vi "receive incidents.vi"(7 "queues":T1, 11 "comms in":T2) -> ()   [LabVIEW 2018]
uses:
  type defs/comms loop data.ctl
  ICL-LabVIEW_General/Incident logger/Incident logger.lvclass
  <vilib>/Modbus/master/Modbus Master.lvclass
  type defs/Queues.ctl
  RT/Type Defs/generic incident.ctl
  RT/Type Defs/warning incident cluster.ctl
  RT/Type Defs/error incident cluster.ctl
  ICL-LabVIEW_General/Incident logger/Incidents/Warning/Warning.lvclass
  C:/Users/cnoon/OneDrive - Imperial College London/LabVIEW/Chris VIs/Incident logger/Incidents/Incident.lvclass
  ICL-LabVIEW_General/Incident logger/Incidents/Message/Message.lvclass
  ICL-LabVIEW_General/Incident logger/Incidents/Error/Error.lvclass
  supporting VIs/polymorphic VIs/enqueue for message handler.vi
  <resource>/objmgr/ni.dex.rc
types:
  T1 = typedef "Queues.ctl" = cluster{"messageHandler":refnum<queue>, "comms":refnum<queue>, "dataStream":refnum<queue>, "dataProcessor":refnum<queue>, "fileIO":refnum<queue>, "userInterface":refnum<queue>, "errors":refnum<queue>, "customCompressor":refnum<queue>}
  T2 = typedef "comms loop data.ctl" = cluster{"params":cluster{"commandStream":cluster{"reader name":string, "writer name":string, "stream buffer size":i32}, "errorStream":cluster{"reader name":string, "writer name":string, "stream buffer size":i32}, "RT IP address":string, "pulserControllerIP":string}, "vars":cluster{"commandStream":refnum<k21>, "Incident logger":refnum<class "Incident logger.lvclass">, "check error scheduled message":u32, "errorStream":refnum<k21>, "watchdogScheduleID":u32, "pulsator":cluster{"pulser connection":refnum<class "Modbus Master.lvclass">, "pulserConnected":bool, "pulsatorScheduleID":u32, "pulserRunning":bool}}}
  T3 = typedef "generic incident.ctl" = cluster{"timestamp":timestamp, "type":string, "Variant":variant}
  T4 = cluster{"Target":string, "Loop":string, "Code":string}
  T5 = typedef "warning incident cluster.ctl" = cluster{"warning description":string, "call chain":string[]}
  T6 = typedef "error incident cluster.ctl" = cluster{"description":string, "call chain":string[], "error":errorcluster}
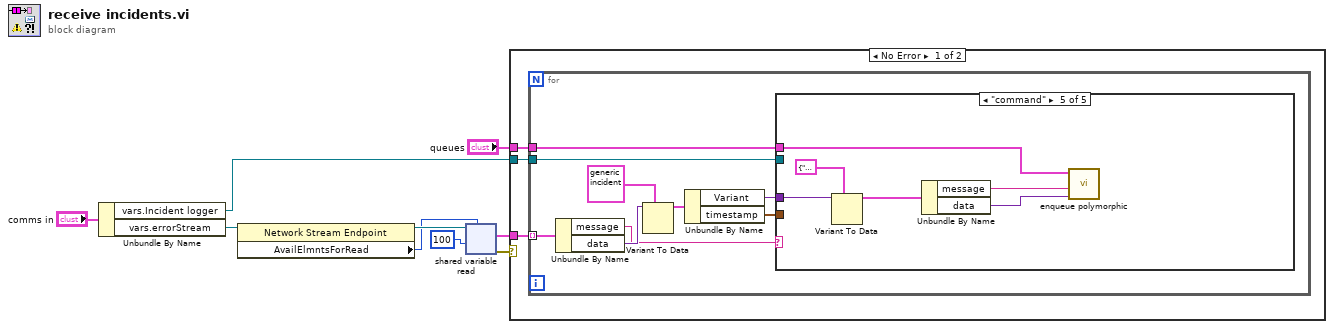
[diagram p0: block diagram]
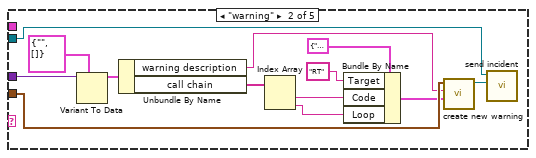
[diagram p3: hidden frame]
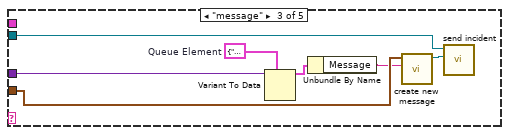
[diagram p4: hidden frame]
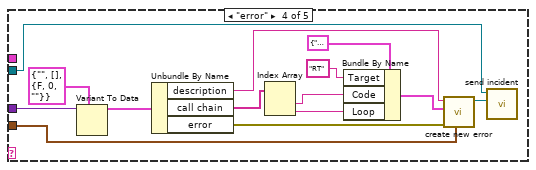
[diagram p5: hidden frame]
diagram:
  n1 = Unbundle By Name("comms in") -> ("vars.Incident logger"=w3:refnum<class "Incident logger.lvclass">, "vars.errorStream"=w8:refnum<k21>)
  n2 = property class="Network Stream Endpoint"(reference=w8) -> (reference out=w7:refnum<k21>, "AvailElmntsForRead"=w6:i32)  [unwired: 1 in, 1 out]
  n3 = shared-variable-read(w7, 100 ("timeout ms (-1)"), w6) -> (w2:errorcluster, w4:cluster{"message":string, "data":variant}[])  [unwired: 1 in, 2 out]
  n4 = case shown="No Error" w2 {
    tunnel: w4 -> [w12 _]
    tunnel: w3 -> [w11 _]
    tunnel: "queues" -> [w10 _]
    frame No Error {
      n5 = for {
        tunnel: w12 -> [w16] mode=indexing
        tunnel: w11 -> [w17]
        tunnel: w10 -> [w13]
        n6 = Unbundle By Name(w16) -> ("message"=w14:string, "data"=w15:variant)
        n7 = Variant To Data(type=T3 {"timestamp"=timestamp(0 s since 1904-01-01), "type"="", "Variant"=variant} ("incident cluster"), Variant=w15) -> (data=w20:T3)  [unwired: 1 in, 1 out]
        n8 = Unbundle By Name(w20) -> ("Variant"=w19:variant, "timestamp"=w18:timestamp)
        n9 = case shown="\"command\"" w14 {
          tunnel: w19 -> [_ w34 w41 w55 w60]
          tunnel: w18 -> [_ w32 w37 w43 _]
          tunnel: w17 -> [_ w22 w39 w48 _]
          tunnel: w13 -> [_ _ _ _ w61]
          frame "", Default {
          }
          frame "warning" {
            n10 = Variant To Data(type=T5 {"warning description"="", "call chain"=[]} ("warning incident"), Variant=w34) -> (data=w31:T5)  [unwired: 1 in, 1 out]
            n11 = Unbundle By Name(w31) -> ("warning description"=w30:string, "call chain"=w26:string[])
            n12 = Index Array(array=w26) -> (element #1=w25:string, element #2=w24:string)  [unwired: 2 in]
            n13 = Bundle By Name(cluster=T4 {"Target"="", "Loop"="", "Code"=""} ("Location"), "Target"="RT", "Code"=w25, "Loop"=w24) -> (w28:T4)
            n14 = call "create new warning.vi"("Location"=w28, "Description"=w30, "set timestamp"=w32) -> ("Warning out"=w23:refnum<class "Warning.lvclass">)  [unwired: 7 in, 1 out]
            n15 = call "send incident.vi"("incident"=w23, "Incident logger in"=w22) -> ()  [unwired: 8 in, 2 out]
          }
          frame "message" {
            w38 = cluster{"Message":string, "Data":variant} {"Message"="", "Data"=variant}  # Queue Element
            n16 = Variant To Data(type=w38, Variant=w41) -> (data=w40:cluster{"Message":string, "Data":variant})  [unwired: 1 in, 1 out]
            n17 = Unbundle By Name(w40) -> ("Message"=w36:string)
            n18 = call "create new message.vi"("Message"=w36, "set timestamp"=w37) -> ("Message"=w35:refnum<class "Message.lvclass">)  [unwired: 8 in, 1 out]
            n19 = call "send incident.vi"("incident"=w35, "Incident logger in"=w39) -> ()  [unwired: 8 in, 2 out]
          }
          frame "error" {
            n20 = Variant To Data(type=T6 {"description"="", "call chain"=[], "error"={"status"=FALSE, "code"=0, "source"=""}} ("error incident"), Variant=w55) -> (data=w54:T6)  [unwired: 1 in, 1 out]
            n21 = Unbundle By Name(w54) -> ("description"=w46:string, "call chain"=w51:string[], "error"=w44:errorcluster)
            n22 = Index Array(array=w51) -> (element #1=w50:string, element #2=w49:string)  [unwired: 2 in]
            n23 = Bundle By Name(cluster=T4 {"Target"="", "Loop"="", "Code"=""} ("Location"), "Target"="RT", "Code"=w50, "Loop"=w49) -> (w45:T4)
            n24 = call "create new error.vi"("set timestamp"=w43, "Error"=w44, "Location"=w45, "Description"=w46) -> ("created error"=w42:refnum<class "Error.lvclass">)  [unwired: 7 in]
            n25 = call "send incident.vi"("incident"=w42, "Incident logger in"=w48) -> ()  [unwired: 8 in, 2 out]
          }
          frame "command" {
            n26 = Variant To Data(type=cluster{"message":string, "data":variant} {"message"="", "data"=variant} ("element"), Variant=w60) -> (data=w58:cluster{"message":string, "data":variant})  [unwired: 1 in, 1 out]
            n27 = Unbundle By Name(w58) -> ("message"=w57:string, "data"=w56:variant)
            n28 = call-poly "enqueue polymorphic.vi"("data"=w56, "message"=w57, "Queues"=w61) -> ()  [unwired: 8 in, 1 out]
          }
        }
      }
    }
    frame Error {
    }
  }
